vi "I2C_UI.vi"() -> ()   [LabVIEW 2023]
doc: "Main VI Of the Application that peroform the I2C Controller"
uses:
  Controls/Button.ctl
  Controls/Customized_Ring.ctl
  Controls/Add_Target_Specification_.ctl
  Controls/Queue_Operation.ctl
  Controls/State_and_Data.ctl
  Controls/I2C_Main_Data.ctl
  Class/I2C/I2C.lvclass
  Controls/Target_Data.ctl
  Controls/Text_File_Operation_Select.ctl
  Controls/UE_Driver_Operation_Select.ctl
  Controls/Converter_Operation_Select.ctl
  Controls/I2C_Data.ctl
  Class/I2C/Controls/Mode.ctl
  Drivers/Queue_Driver/QD_Main.vi
  SubVIs/I2C_to_Target_Spec.vi
  SubVIs/Target_Spec_To_I2C.vi
panel:
  in  "Configure":bool
  out "Tab Control":enum32{"Page 1", "Page 2"}(tab)
  out "Sample_Per_Us":dbl
  out "T_BUF":dbl
  out "T_HD_STA (uS)":dbl
  out "Off_Set (uS)":dbl
  out "Vmax":dbl
  out "Vmin":dbl
  in  "Read_Write":T1 items=["READ", "WRITE"]
  in  "Register_Name":T1
  in  "Target_Name":T1 items=["ADD TARGET"]
  out "Waveform Graph":waveform(dbl)[](graph)
  in  "Data Line":string
  out "History":string
  in  "Error_In":errorcluster
  out "Error_Out":errorcluster
  out "T_HD_DAT (uS)":dbl
  out "T_SU_DAT (uS)":dbl
  out "Frequency (kHz)":dbl
  out "T_SU_STO":dbl
  out "T_Off (uS)":dbl
  out "T_On (uS)":dbl
  in  "Mode":T2
  in  "Update":T2
  in  "Delete":T2
  in  "Target_Select":T1 items=["ADD TARGET"]
  out "Target_Specification":T3 {"Target_Address" format="%x"; "Target_Type" items=["10 Bit Address", "7 Bit Address"]; "T_On (uS)" min=1e-06; "T_Off (uS)" min=1e-06}
  in  "ADD":T2
  # "I2C CONTROLLER"
  # "Target Selection"
  # "History"
  # "Waveform data"
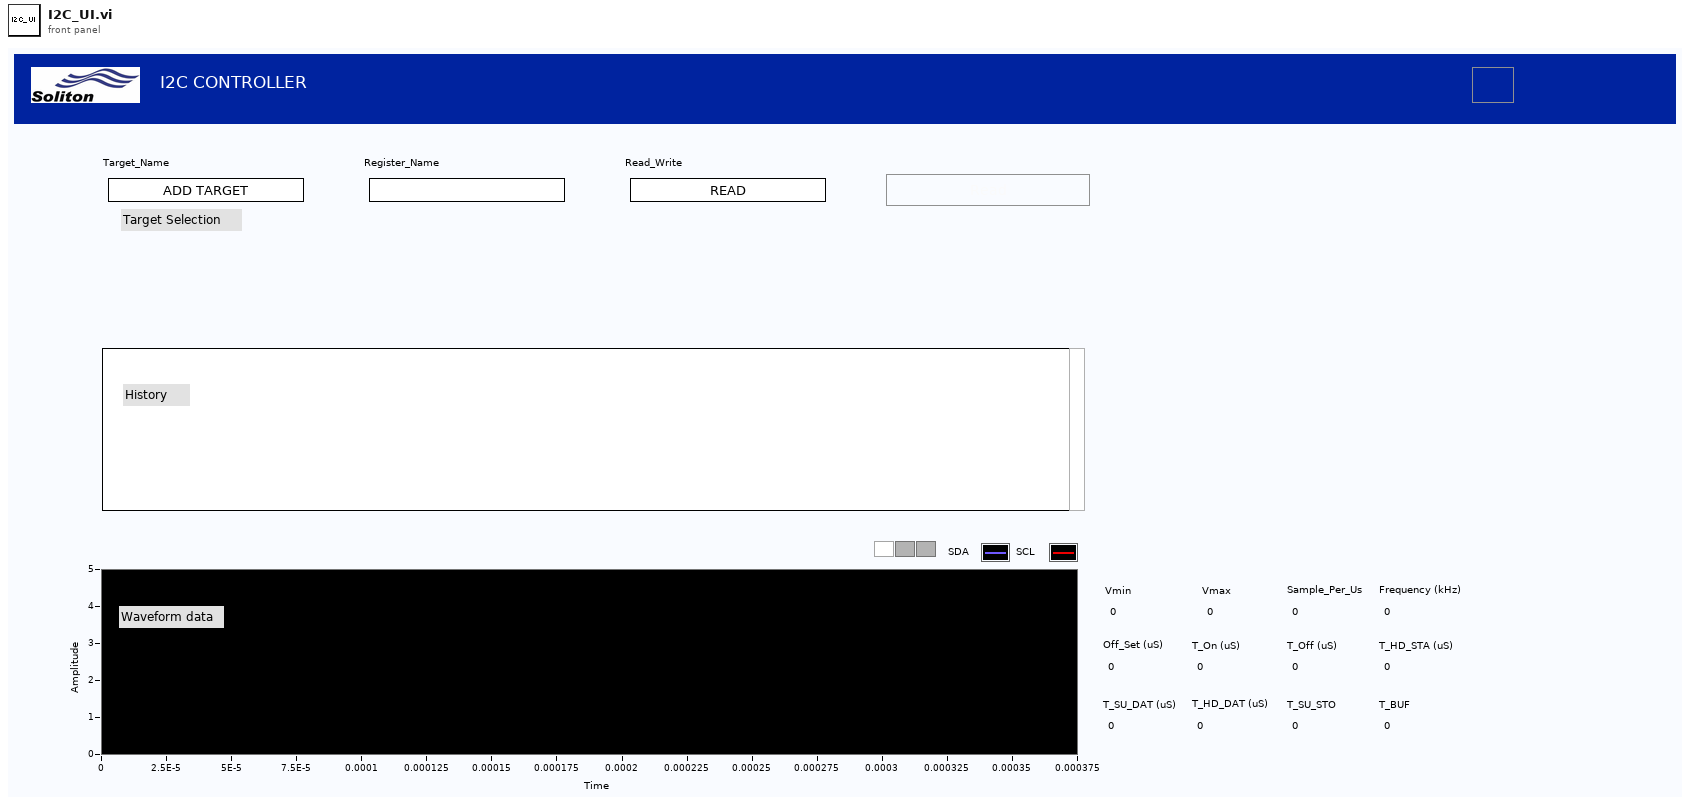
[diagram p1: front panel]
types:
  T1 = typedef "Customized_Ring.ctl" = u16
  T2 = typedef "Button.ctl" = bool
  T3 = typedef "Add_Target_Specification_.ctl" = cluster{"Target_Name":string, "Register_Name":string[], "Register_Address":u16[], "Vmin":dbl, "Vmax":dbl, "Off_Set (uS)":dbl, "T_HD_STA (uS)":dbl, "T_HD_DAT (uS)":dbl, "T_SU_DAT (uS)":dbl, "Frequency (kHz)":dbl, "T_SU_STO":dbl, "T_Off (uS)":dbl, "T_On (uS)":dbl, "T_BUF":dbl, "Sample_Per_Us":dbl, "Target_Type":T1, "Target_Address":u16}
  T4 = typedef "I2C_Main_Data.ctl" = cluster{"Target_Data":map{string, refnum<class "I2C.lvclass">}, "Class_Path":path, "Current_Page":enum32{"Page 1", "Page 2"}, "Class_Names":string[], "I2C_Class":refnum<class "I2C.lvclass">, "Target_Names":string[], "Register_Names":string[], "Selected_Target_Name":string, "Selected_Register_Name":string, "Target_Specification":T5, "Selected_Target_Config":string, "Read_Write":T1, "Add_Target_Reference":refnum<vi>, "Data_Line":string, "I2C_Waveform":waveform(dbl)[], "History":string, "Point_Target_Select":i32, "Ini_File_Path":path, "TVI_Reference":refnum<vi>, "vi reference":refnum<vi>}
  T5 = typedef "Target_Data.ctl" = cluster{"Target_Name":string, "Register_Name":string[], "Register_Address":u16[], "Vmin":dbl, "Vmax":dbl, "Off_Set (uS)":dbl, "T_HD_STA (uS)":dbl, "T_HD_DAT (uS)":dbl, "T_SU_DAT (uS)":dbl, "Frequency (kHz)":dbl, "T_SU_STO":dbl, "T_Off (uS)":dbl, "T_On (uS)":dbl, "T_BUF":dbl, "Sample_Per_Us":dbl, "Target_Type":T1, "Target_Address":u16}
  T6 = typedef "Queue_Operation.ctl" = enum16{"Obtain_Queue", "Enqueue", "Enqueue_First", "Enqueue_N", "Lossy_Enqueue", "Preview", "Queue_Status", "Dequeue", "Flush", "Release_Queue"}
  T7 = typedef "State_and_Data.ctl" = cluster{"State":string, "Data":variant}
  T8 = typedef "I2C_Data.ctl" = cluster{"Vmin":dbl, "Vmax":dbl, "Input":string, "Off_Set (uS)":dbl, "T_HD_STA (uS)":dbl, "Sample_Per_Us":dbl, "T_HD_DAT (uS)":dbl, "T_SU_DAT (uS)":dbl, "Frequency (kHz)":dbl, "T_SU_STO":dbl, "T_Off (uS)":dbl, "T_On (uS)":dbl, "T_BUF":dbl, "Target_Address":u16, "Selected_Register_Address":u8, "Byte_Array":u8[], "Target_Name":string, "Register_Name":string[], "Register_Address":u8[], "Target_Type":T1, "Register_Data":string[]}
  T9 = typedef "UE_Driver_Operation_Select.ctl" = enum16{"Create_UE", "Get_Refnum", "Generate_UE", "Destroy_UE"}
  T10 = typedef "Text_File_Operation_Select.ctl" = enum16{"Initialize", "Read", "Write"}
  T11 = typedef "Converter_Operation_Select.ctl" = enum16{"String_To_Data", "Data_to_String"}
  T12 = typedef "Mode.ctl" = enum16{"Read", "Write"}
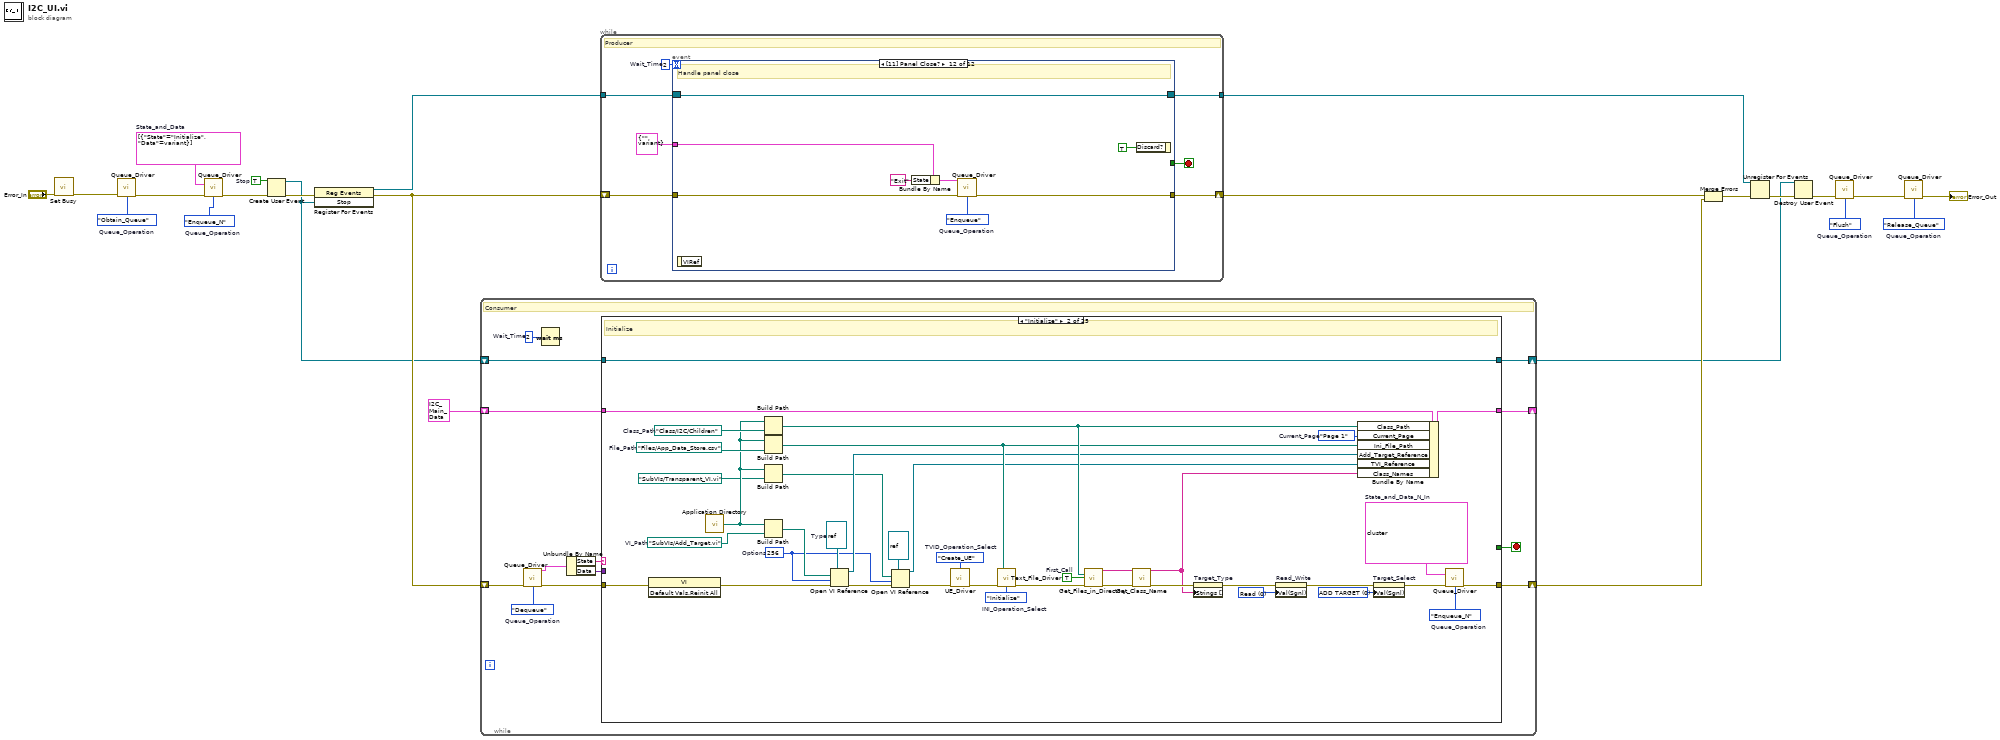
[diagram p0: block diagram]
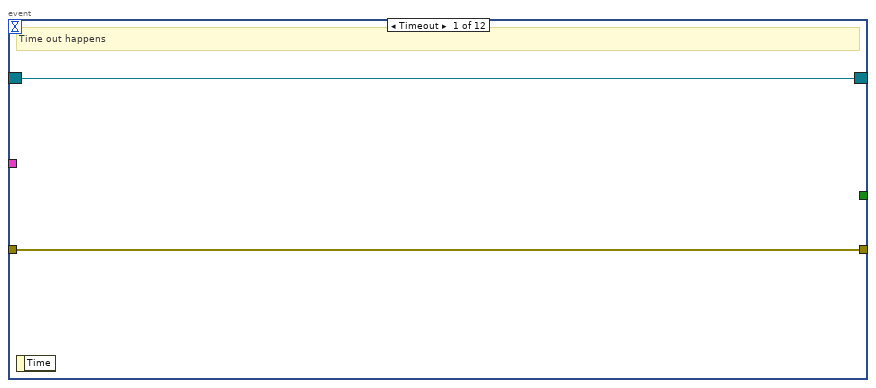
[diagram p2: hidden frame]
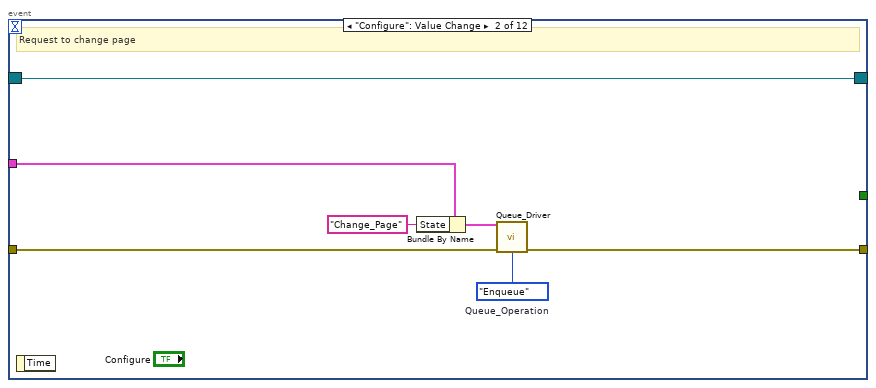
[diagram p3: hidden frame]
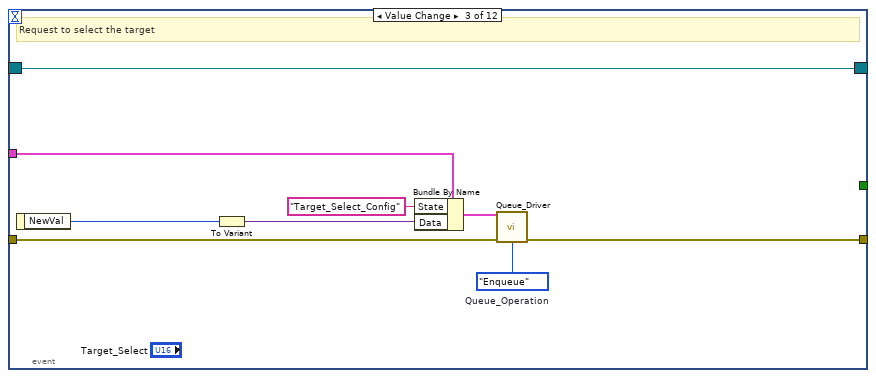
[diagram p4: hidden frame]
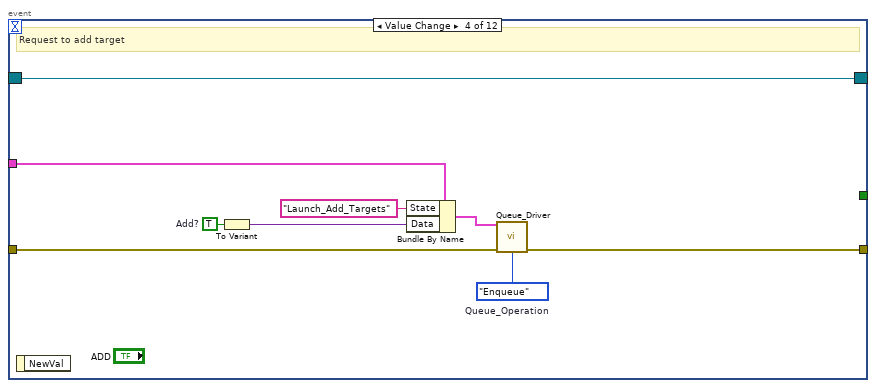
[diagram p5: hidden frame]
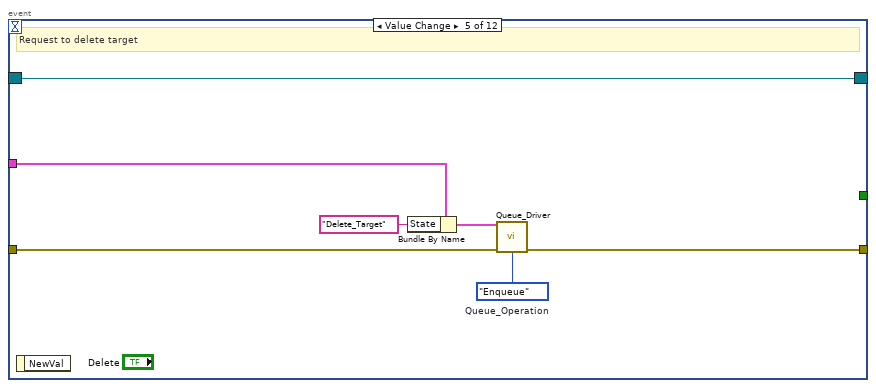
[diagram p6: hidden frame]
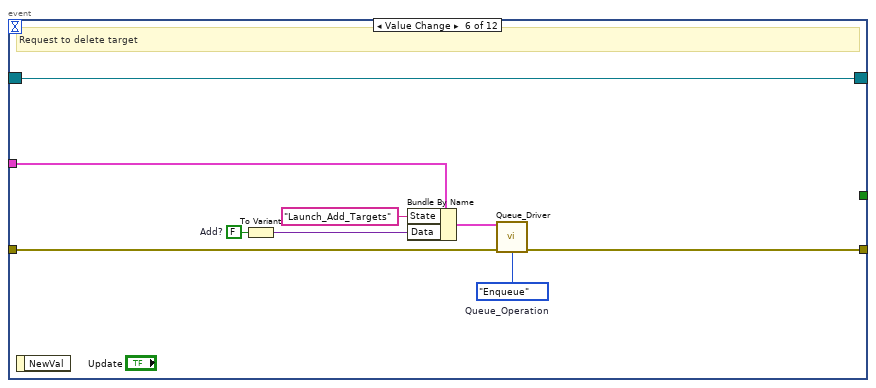
[diagram p7: hidden frame]
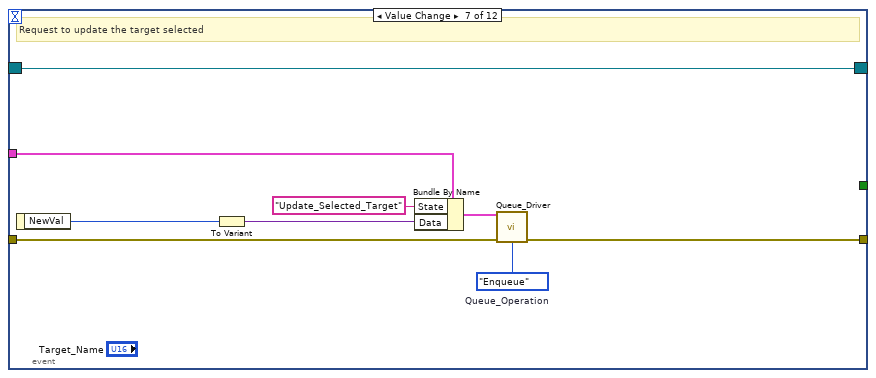
[diagram p8: hidden frame]
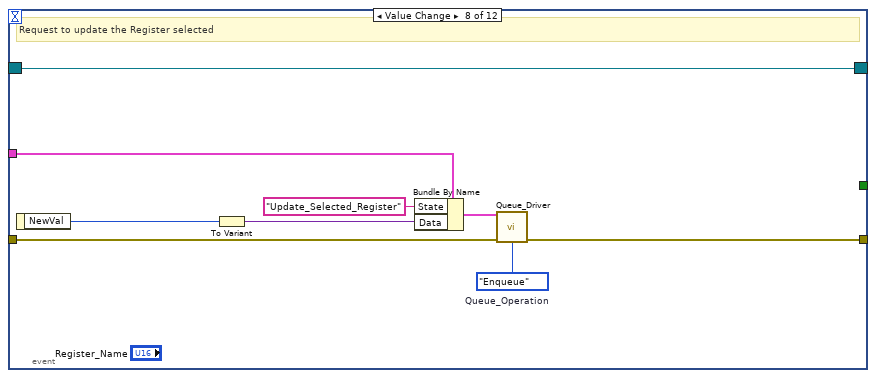
[diagram p9: hidden frame]
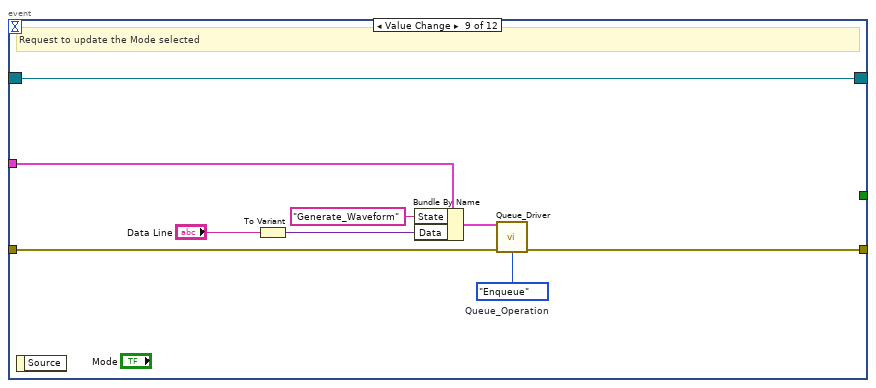
[diagram p10: hidden frame]
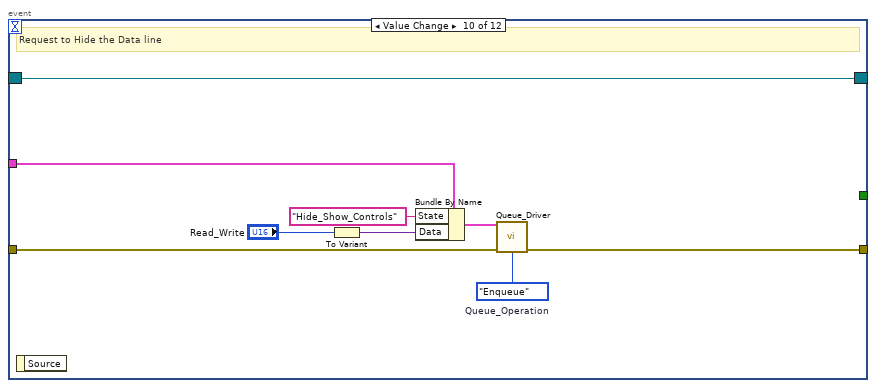
[diagram p11: hidden frame]
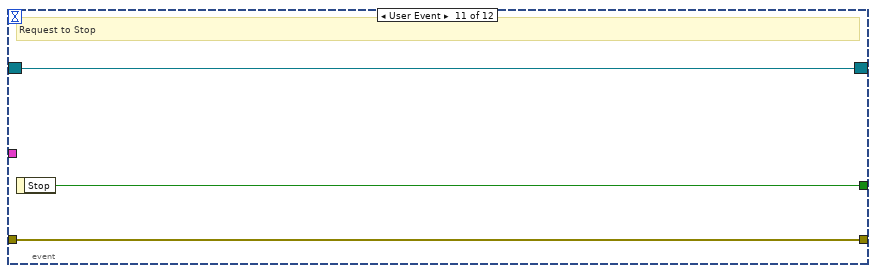
[diagram p12: hidden frame]
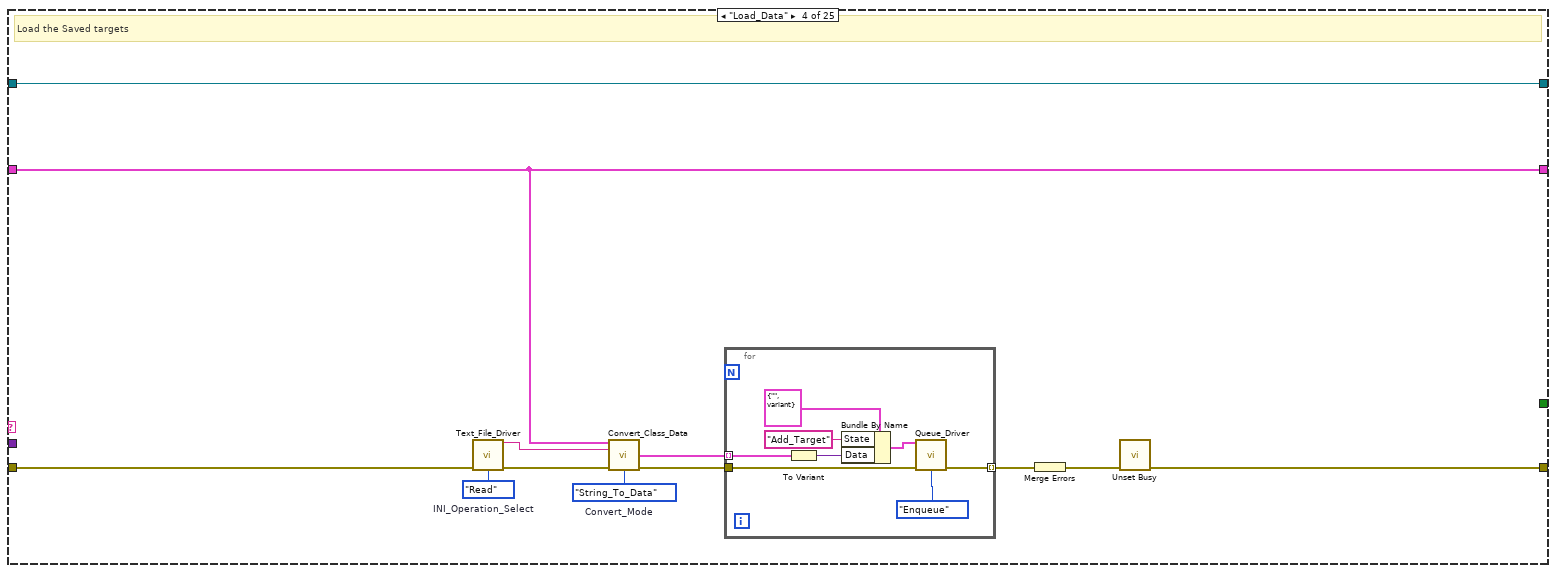
[diagram p15: hidden frame]
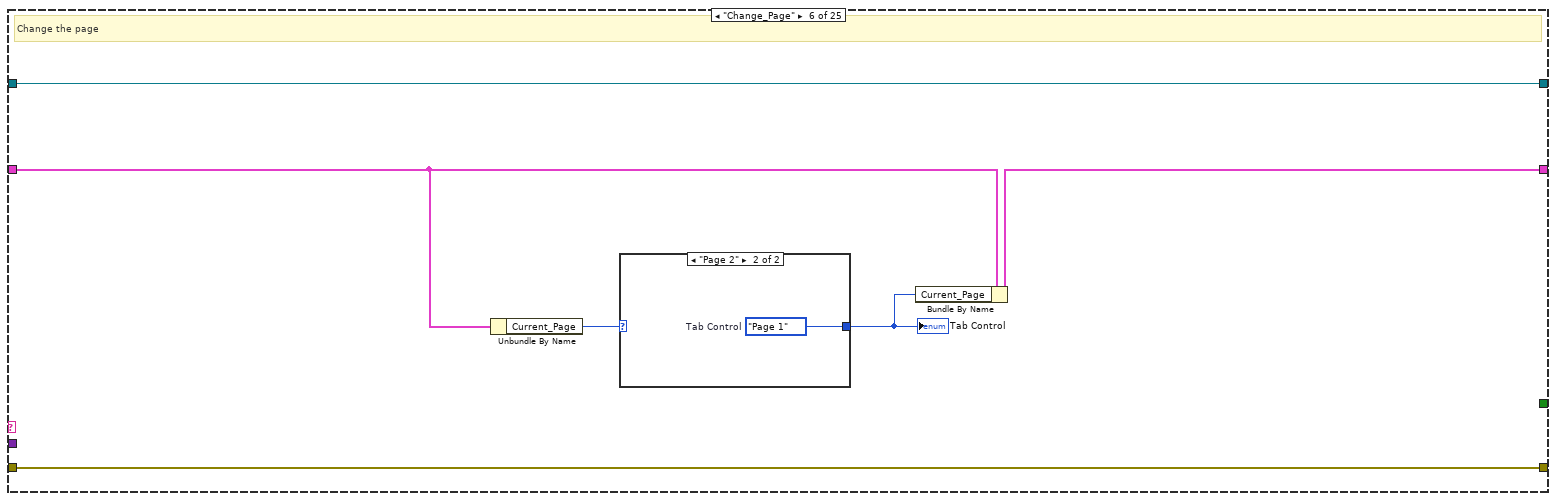
[diagram p17: hidden frame]
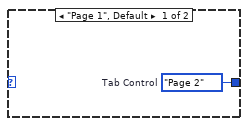
[diagram p18: hidden frame]
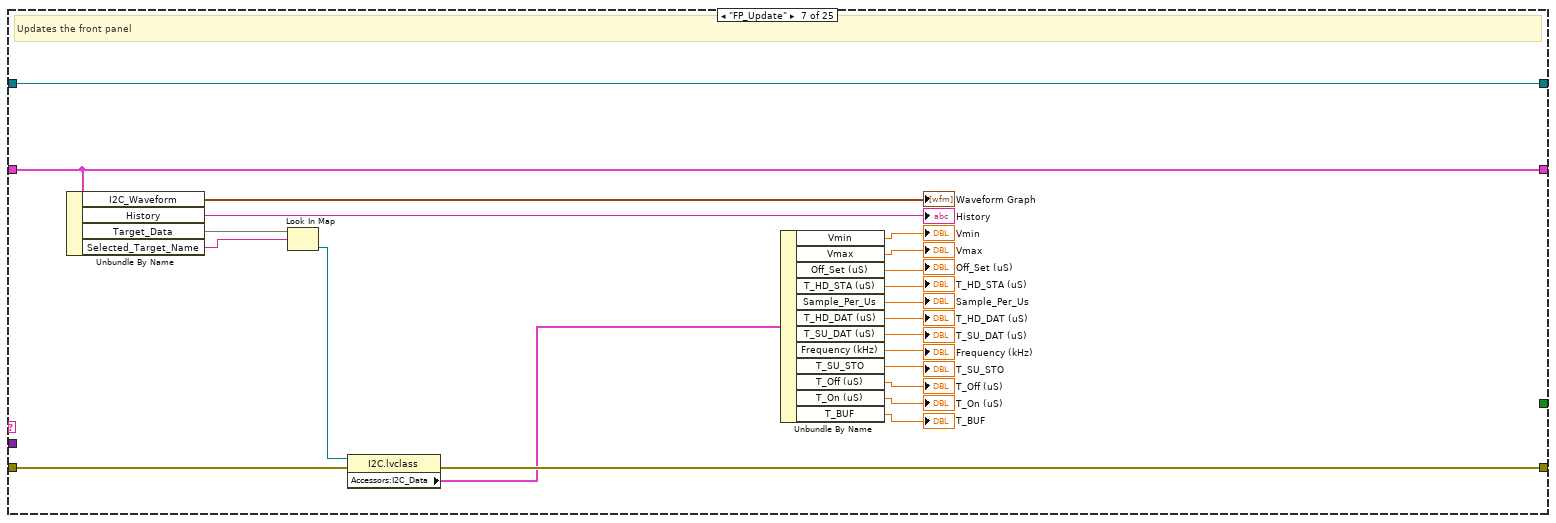
[diagram p19: hidden frame]
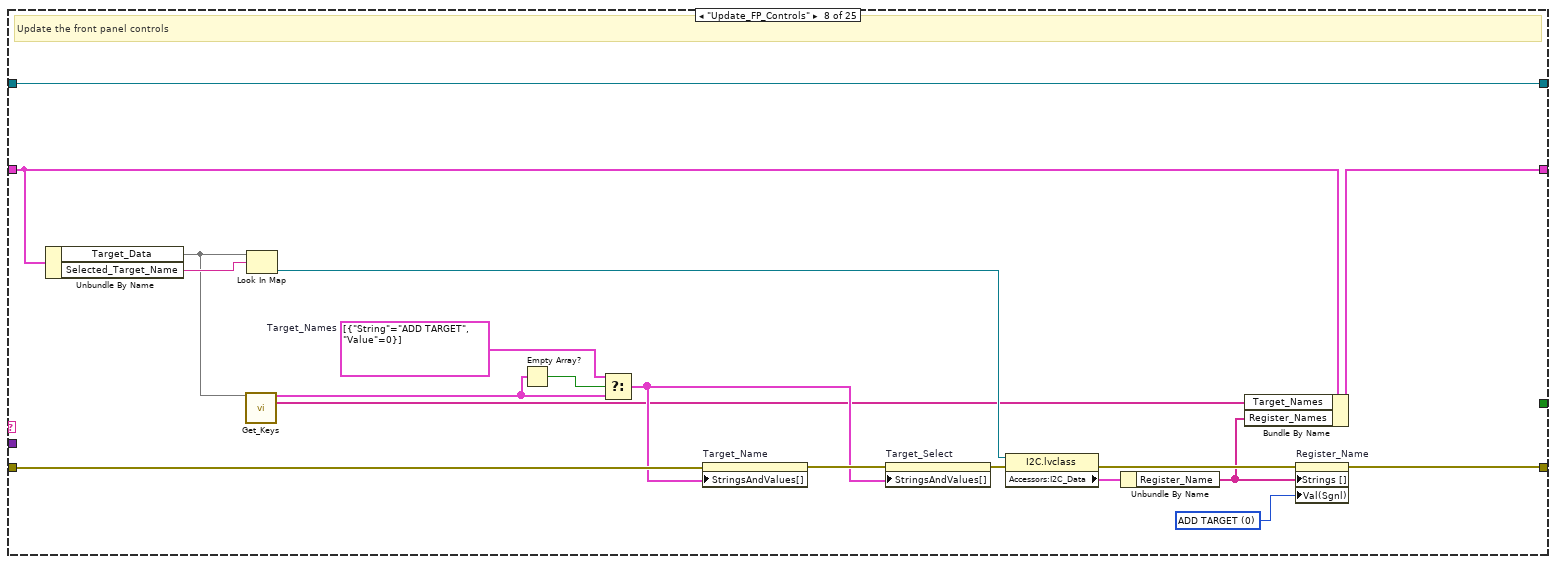
[diagram p20: hidden frame]
diagram:
  w8 = Queue_Operation."Release_Queue"  # Queue_Operation
  w9 = Queue_Operation."Flush"  # Queue_Operation
  w19 = TRUE  # Stop
  w3 = T7[] [{"State"="Initialize", "Data"=variant}]  # State_and_Data
  w22 = Queue_Operation."Enqueue_N"  # Queue_Operation
  w23 = Queue_Operation."Obtain_Queue"  # Queue_Operation
  n1 = call <vilib>:"Set Busy.vi"("error in (no error)"="Error_In") -> ("error out"=w1:errorcluster)  [unwired: 9 in, 1 out]
  n2 = call-poly "Queue_Driver.vi"("Error_In"=w1, "Queue_Operation"=w23) -> ("Error_Out"=w24:errorcluster)  [unwired: 11 in, 2 out]
  n3 = call-poly "Queue_Driver.vi"("State_and_Data_N_In"=w3, "Error_In"=w24, "Queue_Operation"=w22) -> ("Error_Out"=w7:errorcluster)  [unwired: 10 in, 2 out]
  n4 = Create User Event(user event datatype=w19, error in=w7) -> (user event=w4:refnum<user-event>, error out=w20:errorcluster)
  n5 = register-events(error in=w20, w4) -> (reference out=w18:refnum<event-registration>, error out=w5:errorcluster)  [unwired: 1 in]
  n6 = while {
    shift-right: [w29] -> w12
    shift-left: w4 -> [w30]
    shift-right: [w28] -> _
    shift-left: T4 {"Target_Data"={}, "Class_Path"=path "", "Current_Page"=enum."Page 1", "Class_Names"=[], "I2C_Class"=refnum, "Target_Names"=[], "Register_Names"=[], "Selected_Target_Name"="", "Selected_Register_Name"="", "Target_Specification"={"Target_Name"="", "Register_Name"=[], "Register_Address"=[], "Vmin"=0.0, "Vmax"=0.0, "Off_Set (uS)"=0.0, "T_HD_STA (uS)"=0.0, "T_HD_DAT (uS)"=0.0, "T_SU_DAT (uS)"=0.0, "Frequency (kHz)"=0.0, "T_SU_STO"=0.0, "T_Off (uS)"=0.0, "T_On (uS)"=0.0, "T_BUF"=0.0, "Sample_Per_Us"=0.0, "Target_Type"=0, "Target_Address"=0}, "Selected_Target_Config"="", "Read_Write"=0, "Add_Target_Reference"=refnum, "Data_Line"="", "I2C_Waveform"=[], "History"="", "Point_Target_Select"=0, "Ini_File_Path"=path "", "TVI_Reference"=refnum, "vi reference"=refnum} -> [w31]
    shift-right: [w27] -> w16
    shift-left: w5 -> [w37]
    stop <- w26 stop-if-true
    w25 = u32 2  # Wait_Time
    w35 = Queue_Operation."Dequeue"  # Queue_Operation
    # "Consumer"
    n7 = call-poly "Queue_Driver.vi"("Error_In"=w37, "Queue_Operation"=w35) -> ("State_and_Data_Out"=w34:T7, "Error_Out"=w36:errorcluster)  [unwired: 11 in, 1 out]
    n8 = Wait (ms)(milliseconds to wait=w25) -> ()  [unwired: 1 out]
    n9 = Unbundle By Name(w34) -> ("State"=w33:string, "Data"=w32:variant)
    n10 = case shown="\"Initialize\"" w33 {
      tunnel: [w40 w63 w82 w85 w105 w111 w128 w149 w160 w166 w179 w195 w222 w253 w271 w306 w314 w327 w342 w354 w364 w434 w440 w446 w452] -> w27
      tunnel: w36 -> [w40 w78 w82 w84 w105 w111 w135 w148 w161 w177 w192 w195 w201 w256 w279 w306 w326 w337 w351 w354 w367 w437 w440 w448 w461]
      tunnel: w32 -> [_ _ _ _ _ _ _ _ _ w176 _ _ w199 w249 _ _ w323 w334 w349 _ w362 _ _ w449 _]
      tunnel: w31 -> [w39 w56 w81 w89 w104 w109 w133 w153 w157 w175 w190 w194 w229 w252 w277 w305 w324 w335 w345 w353 w366 w435 w439 w447 w458]
      tunnel: [w39 w76 w81 w89 w104 w107 w133 w144 w157 w173 w190 w194 w226 w252 w275 w305 w319 w330 w344 w353 w368 w423 w439 w447 w457] -> w28
      tunnel: w30 -> [w38 w79 w80 w94 w103 w110 w134 w154 w163 w178 w191 w193 w230 w257 w278 w304 w325 w336 w350 w352 w369 w436 w438 w450 w464]
      tunnel: [w38 w79 w80 w94 w103 w110 w134 w154 w163 w178 w191 w193 w230 w257 w278 w304 w325 w336 w350 w352 w369 w436 w438 w450 w463] -> w29
      tunnel: [_ _ _ _ _ _ _ _ _ _ _ _ _ _ _ _ _ _ _ _ _ _ _ _ w462] -> w26
      frame Default {
      }
      frame "Initialize" {
        w41 = T1 0 items=["Read", "Write"] ("Value (Signaling)")
        w52 = UE_Driver_Operation_Select."Create_UE"  # TVID_Operation_Select
        w54 = TRUE  # First_Call
        w58 = T1 0 items=["ADD TARGET"] ("Value (Signaling)")
        w64 = T7[] [{"State"="Update_FP_Controls", "Data"=variant(cluster{"Current_Data":dbl, "Temp_Data":dbl} {"Current_Data"=0.0, "Temp_Data"=0.0})}, {"State"="Config_FP_Update", "Data"=variant(cluster{"Current_Data":dbl, "Temp_Data":dbl} {"Current_Data"=0.0, "Temp_Data"=0.0})}, {"State"="Load_Data", "Data"=variant(cluster{"Current_Data":dbl, "Temp_Data":dbl} {"Current_Data"=0.0, "Temp_Data"=0.0})}]  # State_and_Data_N_In
        w65 = Queue_Operation."Enqueue_N"  # Queue_Operation
        w67 = Text_File_Operation_Select."Initialize"  # INI_Operation_Select
        w68 = path "Files/App_Data_Store.csv"  # File_Path
        w69 = refnum<vi> refnum  # Type
        w43 = 256  # Options
        w72 = path "SubVIs/Add_Target.vi"  # VI_Path
        w74 = enum32{"Page 1", "Page 2"}."Page 1"  # Current_Page
        w77 = path "Class/I2C/Children"  # Class_Path
        # "Initialize"
        n11 = invoke class="VI" method="Default Vals.Reinit All"(error in=w78) -> (error out=w70:errorcluster)  [unwired: 2 in, 2 out]
        n12 = call <vilib>:"Application Directory.vi"() -> ("Application Directory"=w50:path)
        n13 = Build Path(base path=w50, name or relative path=w77) -> (appended path=w66:path)
        n14 = Build Path(base path=w50, name or relative path=w68) -> (appended path=w62:path)
        n15 = Build Path(base path=w50, name or relative path=path "SubVIs/Transparent_VI.vi") -> (appended path=w46:path)
        n16 = Build Path(base path=w50, name or relative path=w72) -> (appended path=w71:path)
        n17 = Open VI Reference(type specifier VI Refnum (for type only)=w69, vi path=w71, options=w43, error in (no error)=w70) -> (vi reference=w51:refnum<vi>, error out=w48:errorcluster)  [unwired: 2 in]
        n18 = Open VI Reference(type specifier VI Refnum (for type only)=refnum<vi> refnum, vi path=w46, options=w43, error in (no error)=w48) -> (vi reference=w44:refnum<vi>, error out=w47:errorcluster)  [unwired: 2 in]
        n19 = call "UE_Driver.vi"("TVID_Operation_Select"=w52, "Error_In"=w47) -> ("Error_Out"=w53:errorcluster)  [unwired: 11 in, 2 out]
        n20 = call "Text_File_Driver.vi"("Config_File_Path"=w62, "Error_Out"=w53, "INI_Operation_Select"=w67) -> ("Error_Out"=w57:errorcluster)  [unwired: 11 in, 1 out]
        n21 = call "Get_Files_in_Directory.vi"("File_Path"=w66, "First_Call"=w54, "Error_In"=w57) -> ("File_Names_Out"=w75:string[], "Error_Out"=w61:errorcluster)  [unwired: 11 in]
        n22 = call "Get_Class_Name.vi"("File_Names"=w75, "Error_In"=w61) -> ("Class_Names"=w60:string[], "Error_Out"=w73:errorcluster)  [unwired: 12 in]
        n23 = property on="Target_Type" class="Ring (strict)"(error in=w73, "Strings []"=w60) -> (error out=w55:errorcluster)  [unwired: 1 in, 1 out]
        n24 = property on="Read_Write" class="Ring (strict)"(error in=w55, "Val(Sgnl)"=w41) -> (error out=w42:errorcluster)  [unwired: 1 in, 1 out]
        n25 = Bundle By Name(cluster=w56, "Class_Path"=w66, "Current_Page"=w74, "Ini_File_Path"=w62, "Add_Target_Reference"=w51, "TVI_Reference"=w44, "Class_Names"=w60) -> (w76:T4)
        n26 = property on="Target_Select" class="Ring (strict)"(error in=w42, "Val(Sgnl)"=w58) -> (error out=w59:errorcluster)  [unwired: 1 in, 1 out]
        n27 = call-poly "Queue_Driver.vi"("State_and_Data_N_In"=w64, "Error_In"=w59, "Queue_Operation"=w65) -> ("Error_Out"=w63:errorcluster)  [unwired: 10 in, 2 out]
      }
      frame "---------------------Setup_States------------------" {
      }
      frame "Load_Data" {
        w90 = Converter_Operation_Select."String_To_Data"  # Convert_Mode
        w93 = Text_File_Operation_Select."Read"  # INI_Operation_Select
        # "Load the Saved targets"
        n28 = call "Text_File_Driver.vi"("Error_Out"=w84, "INI_Operation_Select"=w93) -> ("Data_Out"=w91:string, "Error_Out"=w92:errorcluster)  [unwired: 12 in]
        n29 = call "Convert_Class_Data.vi"("I2C_Data"=w89, "CSV_String_In"=w91, "Error_In"=w92, "Convert_Mode"=w90) -> ("Data"=w83:T8[], "Error_Out"=w87:errorcluster)  [unwired: 8 in, 2 out]
        n30 = for {
          tunnel: [w102] -> w88 mode=indexing
          tunnel: w83 -> [w98] mode=indexing
          tunnel: w87 -> [w95]
          n31 = To Variant(anything=w98) -> (Variant=w97:variant)
          n32 = Bundle By Name(cluster=T7 {"State"="", "Data"=variant} ("State_and_Data_In"), "State"="Add_Target", "Data"=w97) -> (w99:T7)
          n33 = call-poly "Queue_Driver.vi"("State_and_Data_In"=w99, "Error_In"=w95, "Queue_Operation"=Queue_Operation."Enqueue") -> ("Error_Out"=w102:errorcluster)  [unwired: 10 in, 2 out]
        }
        n34 = Merge Errors(w88) -> (w86:errorcluster)
        n35 = call <vilib>:"Unset Busy.vi"("error in (no error)"=w86) -> ("error out"=w85:errorcluster)  [unwired: 10 in]
      }
      frame "-----------------Front_Panel_Updates--------------" {
      }
      frame "Change_Page" {
        # "Change the page"
        n36 = Unbundle By Name(w109) -> ("Current_Page"=w108:enum32{"Page 1", "Page 2"})
        n37 = case shown="\"Page 2\"" w108 {
          tunnel: [w112 w113] -> w106
          frame "Page 1", Default {
            w112 = enum32{"Page 1", "Page 2"}."Page 2"  # Tab Control
          }
          frame "Page 2" {
            w113 = enum32{"Page 1", "Page 2"}."Page 1"  # Tab Control
          }
        }
        "Tab Control" <- w106
        n38 = Bundle By Name(cluster=w109, "Current_Page"=w106) -> (w107:T4)
      }
      frame "FP_Update" {
        # "Updates the front panel"
        n39 = Unbundle By Name(w133) -> ("I2C_Waveform"=→"Waveform Graph":waveform(dbl)[], "History"=→"History":string, "Target_Data"=w130:map{string, refnum<class "I2C.lvclass">}, "Selected_Target_Name"=w129:string)
        n40 = Look In Map(map=w130, key=w129) -> (value=w127:refnum<class "I2C.lvclass">)  [unwired: 1 in, 1 out]
        n41 = property class="I2C.lvclass"(reference=w127, error in=w135) -> (error out=w128:errorcluster, "Accessors:I2C_Data"=w126:T8)  [unwired: 1 out]
        n42 = Unbundle By Name(w126) -> ("Vmin"=→"Vmin":dbl, "Vmax"=→"Vmax":dbl, "Off_Set (uS)"=→"Off_Set (uS)":dbl, "T_HD_STA (uS)"=→"T_HD_STA (uS)":dbl, "Sample_Per_Us"=→"Sample_Per_Us":dbl, "T_HD_DAT (uS)"=→"T_HD_DAT (uS)":dbl, "T_SU_DAT (uS)"=→"T_SU_DAT (uS)":dbl, "Frequency (kHz)"=→"Frequency (kHz)":dbl, "T_SU_STO"=→"T_SU_STO":dbl, "T_Off (uS)"=→"T_Off (uS)":dbl, "T_On (uS)"=→"T_On (uS)":dbl, "T_BUF"=→"T_BUF":dbl)
      }
      frame "Update_FP_Controls" {
        w136 = T1 0 items=["ADD TARGET"] ("Value (Signaling)")
        w141 = cluster{"String":string, "Value":u16}[] [{"String"="ADD TARGET", "Value"=0}]  # Target_Names
        # "Update the front panel controls"
        n43 = Unbundle By Name(w153) -> ("Target_Data"=w140:map{string, refnum<class "I2C.lvclass">}, "Selected_Target_Name"=w146:string)
        n44 = call "Get_Keys.vi"("Target_Data"=w140) -> ("Keys_and_Index"=w139:cluster{"String":string, "Value":u16}[], "Keys"=w137:string[])  [unwired: 10 in, 3 out]
        n45 = Look In Map(map=w140, key=w146) -> (value=w151:refnum<class "I2C.lvclass">)  [unwired: 1 in, 1 out]
        n46 = Empty Array?(array=w139) -> (empty?=w142:bool)
        n47 = Select(t=w141, s=w142, f=w139) -> (s? t:f=w138:cluster{"String":string, "Value":u16}[])
        n48 = property on="Target_Name" class="Ring (strict)"(error in=w148, "StringsAndValues[]"=w138) -> (error out=w147:errorcluster)  [unwired: 1 in, 1 out]
        n49 = property on="Target_Select" class="Ring (strict)"(error in=w147, "StringsAndValues[]"=w138) -> (error out=w145:errorcluster)  [unwired: 1 in, 1 out]
        n50 = property class="I2C.lvclass"(reference=w151, error in=w145) -> (error out=w152:errorcluster, "Accessors:I2C_Data"=w150:T8)  [unwired: 1 out]
        n51 = Unbundle By Name(w150) -> ("Register_Name"=w143:string[])
        n52 = Bundle By Name(cluster=w153, "Target_Names"=w137, "Register_Names"=w143) -> (w144:T4)
        n53 = property on="Register_Name" class="Ring (strict)"(error in=w152, "Strings []"=w143, "Val(Sgnl)"=w136) -> (error out=w149:errorcluster)  [unwired: 1 in, 1 out]
      }
      frame "Config_FP_Update" {
        # "Updates the config panel display"
        n54 = Unbundle By Name(w157) -> ("Target_Data"=w158:map{string, refnum<class "I2C.lvclass">}, "Selected_Target_Config"=w159:string)
        n55 = Look In Map(map=w158, key=w159) -> (value=w162:refnum<class "I2C.lvclass">)  [unwired: 1 in, 1 out]
        n56 = property class="I2C.lvclass"(reference=w162, error in=w161) -> (error out=w160:errorcluster, "Accessors:I2C_Data"=w156:T8)  [unwired: 1 out]
        n57 = call-poly "Converter.vi"("I2C_Data"=w156) -> ("Target_Specification"=→"Target_Specification":T3)  [unwired: 14 in]
      }
      frame "Hide_Show_Controls" {
        w170 = "Write"  # Text
        w171 = "Read"  # Text
        # "Hide and show the data line in read and write mode respectively"
        n58 = Unbundle By Name(w175) -> ("Read_Write"=w174:T1)
        n59 = Variant To Data(error in=w177, type=w174, Variant=w176) -> (data=w168:T1, error out=w169:errorcluster)
        n60 = Bundle By Name(cluster=w175, "Read_Write"=w168) -> (w173:T4)
        n61 = Not Equal To 0?(x=w168) -> (x != 0?=w164:bool)
        n62 = property on="Data Line" class="Str"(error in=w169, "Visible"=w164, "Value"="", "Key Focus"=w164) -> (error out=w167:errorcluster)  [unwired: 1 in, 1 out]
        n63 = Select(t=w170, s=w164, f=w171) -> (s? t:f=w172:string)
        n64 = property on="Mode" class="Bool (strict)"(error in=w167, "BoolText.Text"=w172) -> (error out=w166:errorcluster)  [unwired: 1 in, 1 out]
      }
      frame "Point_Target_Select" {
        w185 = T1 0 items=["ADD TARGET"]  # Type
        w188 = 0  # Index
        # "Makes the controls point valid values"
        n65 = Unbundle By Name(w190) -> ("Selected_Target_Name"=w182:string, "Target_Data"=w183:map{string, refnum<class "I2C.lvclass">})  [unwired: 1 out]
        n66 = call "Get_Keys.vi"("Target_Data"=w183) -> ("Keys"=w181:string[])  [unwired: 10 in, 4 out]
        n67 = Search 1D Array(1D array=w181, element=w182) -> (index of element=w180:i32)  [unwired: 1 in]
        n68 = Greater Or Equal To 0?(x=w180) -> (x >= 0?=w187:bool)
        n69 = Select(t=w180, s=w187, f=w188) -> (s? t:f=w186:i32)
        n70 = Coerce To Type(0:w186, 1:w185) -> (2:w184:T1)
        n71 = property on="Target_Select" class="Ring (strict)"(error in=w192, "Val(Sgnl)"=w184) -> (error out=w189:errorcluster)  [unwired: 1 in, 1 out]
        n72 = property on="Target_Name" class="Ring (strict)"(error in=w189, "Val(Sgnl)"=w184) -> (error out=w179:errorcluster)  [unwired: 1 in, 1 out]
      }
      frame "--------------------Manage_Targets---------------" {
      }
      frame "Add_Target" {
        w206 = T7[] [{"State"="Update_FP_Controls", "Data"=variant(cluster{"Current_Data":dbl, "Temp_Data":dbl} {"Current_Data"=0.0, "Temp_Data"=0.0})}, {"State"="Config_FP_Update", "Data"=variant(cluster{"Current_Data":dbl, "Temp_Data":dbl} {"Current_Data"=0.0, "Temp_Data"=0.0})}, {"State"="Point_Target_Select", "Data"=variant(cluster{"Current_Data":dbl, "Temp_Data":dbl} {"Current_Data"=0.0, "Temp_Data"=0.0})}]  # State_and_Data_N_In
        w207 = Queue_Operation."Enqueue_N"  # Queue_Operation
        w208 = 0  # Type
        w221 = "%s\\\\%s\\\\%s.lvclass"  # Format_String
        # "Add targets and populate into controls"
        n73 = Unbundle By Name(w229) -> ("Target_Names"=w224:string[], "Target_Data"=w225:map{string, refnum<class "I2C.lvclass">}, "I2C_Class"=w227:refnum<class "I2C.lvclass">, "Class_Path"=w228:path, "Class_Names"=w223:string[])
        n74 = Variant To Data(error in=w201, type=T8 {"Vmin"=0.0, "Vmax"=1.0, "Input"="", "Off_Set (uS)"=0.0, "T_HD_STA (uS)"=0.0, "Sample_Per_Us"=0.0, "T_HD_DAT (uS)"=0.0, "T_SU_DAT (uS)"=0.0, "Frequency (kHz)"=0.0, "T_SU_STO"=0.0, "T_Off (uS)"=0.0, "T_On (uS)"=0.0, "T_BUF"=0.0, "Target_Address"=0, "Selected_Register_Address"=0, "Byte_Array"=[], "Target_Name"="", "Register_Name"=[], "Register_Address"=[], "Target_Type"=0, "Register_Data"=[]} ("I2C_Data"), Variant=w199) -> (data=w197:T8, error out=w200:errorcluster)
        n75 = Unbundle By Name(w197) -> ("Register_Name"=w198:string[], "Target_Name"=w205:string, "Target_Type"=w211:T1)
        n76 = Coerce To Type(0:w211, 1:w208) -> (2:w209:i32)
        n77 = Index Array(array=w223, index=w209) -> (element=w210:string)
        n78 = Format Into String(format string=w221, error in=w200, w228, w210, w210) -> (resulting string=w220:string, error out=w219:errorcluster)  [unwired: 1 in]
        n79 = String To Path(string=w220) -> (path=w217:path)
        n80 = call <vilib>:"Get LV Class Default Value.vi"("error in (no error)"=w219, "class path"=w217) -> ("error out"=w218:errorcluster, "object"=w215:refnum<class>)  [unwired: 8 in]
        n81 = To More Specific Class(target class=w227, reference=w215, error in=w218) -> (specific class reference=w214:refnum<class "I2C.lvclass">, error out=w216:errorcluster)
        n82 = property class="I2C.lvclass"(reference=w214, error in=w216, "Accessors:I2C_Data"=w197) -> (reference out=w212:refnum<class "I2C.lvclass">, error out=w203:errorcluster)
        n83 = Insert Into Array(array=w224, new element=w205) -> (w202:string[])  [unwired: 1 in]
        n84 = Insert Into Map(map in=w225, key=w205, value=w212) -> (map out=w213:map{string, refnum<class "I2C.lvclass">})  [unwired: 2 out]
        n85 = Index Array(array=w198) -> (element=w204:string)  [unwired: 1 in]
        n86 = Bundle By Name(cluster=w229, "Selected_Target_Name"=w205, "Target_Names"=w202, "Selected_Target_Config"=w205, "Target_Data"=w213, "Selected_Register_Name"=w204) -> (w226:T4)
        n87 = call-poly "Queue_Driver.vi"("State_and_Data_N_In"=w206, "Error_In"=w203, "Queue_Operation"=w207) -> ("Error_Out"=w222:errorcluster)  [unwired: 10 in, 2 out]
      }
      frame "Launch_Add_Targets" {
        w232 = UE_Driver_Operation_Select."Generate_UE"  # TVID_Operation_Select
        w242 = T8 {"Vmin"=0.0, "Vmax"=5.0, "Input"="", "Off_Set (uS)"=10.0, "T_HD_STA (uS)"=5.0, "Sample_Per_Us"=1000.0, "T_HD_DAT (uS)"=5.0, "T_SU_DAT (uS)"=0.25, "Frequency (kHz)"=0.0, "T_SU_STO"=4.0, "T_Off (uS)"=5.0, "T_On (uS)"=5.0, "T_BUF"=5.0, "Target_Address"=0, "Selected_Register_Address"=0, "Byte_Array"=[], "Target_Name"="", "Register_Name"=[], "Register_Address"=[], "Target_Type"=0, "Register_Data"=[]}  # Empty_I2C
        # "Launch the add target page to add or edit the targets"
        n88 = Unbundle By Name(w252) -> ("Add_Target_Reference"=w238:refnum<vi>, "TVI_Reference"=w234:refnum<vi>, "Target_Data"=w247:map{string, refnum<class "I2C.lvclass">}, "Selected_Target_Name"=w246:string)
        n89 = Variant To Data(error in=w256, type=FALSE, Variant=w249) -> (data=w243:bool, error out=w250:errorcluster)
        n90 = Look In Map(map=w247, key=w246) -> (value=w245:refnum<class "I2C.lvclass">)  [unwired: 1 in, 1 out]
        n91 = property class="I2C.lvclass"(reference=w245, error in=w250) -> (error out=w237:errorcluster, "Accessors:I2C_Data"=w244:T8)  [unwired: 1 out]
        n92 = Select(t=w242, s=w243, f=w244) -> (s? t:f=w240:T8)
        n93 = call-poly "Converter.vi"("I2C_Data"=w240) -> ("Target_Specification"=w231:T3)  [unwired: 14 in]
        n94 = call-by-ref "Start Asynchronous Call"(reference=w234, error in=w237) -> (error out=w235:errorcluster)  [unwired: 19 in, 2 out]
        n95 = call-by-ref "?"(reference=w238, error in=w235, "Data"=w231) -> (error out=w236:errorcluster, "Target_Specification_Out"=w239:T3, "Add?"=w251:bool, "Error_Out"=w254:errorcluster)  [unwired: 12 in, 1 out]
        n96 = call "UE_Driver.vi"("TVID_Operation_Select"=w232, "Error_In"=w236) -> ("Error_Out"=w233:errorcluster)  [unwired: 11 in, 2 out]
        n97 = Merge Errors(w233, w254) -> (w255:errorcluster)
        n98 = call-poly "Converter.vi"("Input_Data"=w239) -> ("I2C_Data"=w241:T8)  [unwired: 14 in]
        n99 = case shown="False" w251 {
          tunnel: w255 -> [w265 w266]
          tunnel: [w264 w266] -> w253
          tunnel: w241 -> [w259 _]
          frame False {
            w263 = Queue_Operation."Enqueue"  # Queue_Operation
            # "Add if added"
            n100 = To Variant(anything=w259) -> (Variant=w258:variant)
            n101 = Bundle By Name(cluster=T7 {"State"="", "Data"=variant} ("State_and_Data_In"), "State"="Add_Target", "Data"=w258) -> (w261:T7)
            n102 = call-poly "Queue_Driver.vi"("State_and_Data_In"=w261, "Error_In"=w265, "Queue_Operation"=w263) -> ("Error_Out"=w264:errorcluster)  [unwired: 10 in, 2 out]
          }
          frame True {
            # "Dont add if canceled"
          }
        }
      }
      frame "Delete_Target" {
        w272 = "%s"  # Format_String
        w274 = "Do you want to delete "  # Initial_Message
        # "Delete the targets"
        n103 = Unbundle By Name(w277) -> ("Target_Names"=w269:string[], "Target_Data"=w276:map{string, refnum<class "I2C.lvclass">}, "Selected_Target_Config"=w273:string)
        n104 = Empty Array?(array=w269) -> (empty?=w268:bool)
        n105 = Format Into String(format string=w272, initial string=w274, error in=w279, w273) -> (resulting string=w267:string, error out=w270:errorcluster)
        n106 = case shown="False" w268 {
          tunnel: w277 -> [w283 w303]
          tunnel: w276 -> [w299 _]
          tunnel: [w284 w303] -> w275
          tunnel: w273 -> [w294 _]
          tunnel: [w296 w302] -> w271
          tunnel: w270 -> [w290 w302]
          tunnel: w267 -> [w286 _]
          frame False {
            w288 = "No"  # Dont
            w287 = "Yes"  # Delete
            w291 = T7[] [{"State"="Update_FP_Controls", "Data"=variant(cluster{"Current_Data":dbl, "Temp_Data":dbl} {"Current_Data"=0.0, "Temp_Data"=0.0})}, {"State"="Point_Target_Select", "Data"=variant(cluster{"Current_Data":dbl, "Temp_Data":dbl} {"Current_Data"=0.0, "Temp_Data"=0.0})}, {"State"="Config_FP_Update", "Data"=variant(cluster{"Current_Data":dbl, "Temp_Data":dbl} {"Current_Data"=0.0, "Temp_Data"=0.0})}]  # State_and_Data_N_In
            w295 = Queue_Operation."Enqueue_N"  # Queue_Operation
            # "Delete if target exist"
            n107 = Unbundle By Name(w283) -> ("Target_Names"=w293:string[])
            n108 = Remove From Map(10:w294, 11:w299) -> (3:w297:map{string, refnum<class "I2C.lvclass">})  [unwired: 2 out]
            n109 = Search 1D Array(1D array=w293, element=w294) -> (index of element=w289:i32)  [unwired: 1 in]
            n110 = Two Button Dialog(message=w286, 1:w288, 2:w287) -> (T button?=w282:bool)
            n111 = Delete From Array(array=w293, index=w289) -> (array with subset deleted=w292:string[])  [unwired: 1 in, 1 out]
            n112 = Bundle By Name(cluster=w283, "Target_Names"=w292, "Target_Data"=w297) -> (w298:T4)
            n113 = Not(x=w282) -> (.not. x?=w280:bool)
            n114 = Select(t=w283, s=w280, f=w298) -> (s? t:f=w284:T4)
            n115 = Select(t=T7[] [] ("f"), s=w280, f=w291) -> (s? t:f=w285:T7[])
            n116 = call-poly "Queue_Driver.vi"("State_and_Data_N_In"=w285, "Error_In"=w290, "Queue_Operation"=w295) -> ("Error_Out"=w296:errorcluster)  [unwired: 10 in, 2 out]
          }
          frame True {
            w300 = "Ok"  # Ack
            w301 = "No targets to delete"  # Message
            # "Prompt user if there is no target"
            n117 = One Button Dialog(message=w301, button name ("OK")=w300) -> ()  [unwired: 1 out]
          }
        }
      }
      frame "----------------- Manage_States_Data---------------" {
      }
      frame "Update_Selected_Target" {
        w316 = Queue_Operation."Enqueue"  # Queue_Operation
        w317 = T7 {"State"="Update_FP_Controls", "Data"=variant}  # State_and_Data_In
        w322 = u16 0  # Type
        # "Update selected target"
        n118 = Unbundle By Name(w324) -> ("Target_Data"=w313:map{string, refnum<class "I2C.lvclass">}, "Target_Names"=w321:string[])
        n119 = Variant To Data(error in=w326, type=w322, Variant=w323) -> (data=w320:u16, error out=w315:errorcluster)
        n120 = To Long Integer(number=w320) -> (32bit integer=w318:i32)
        n121 = Index Array(array=w321, index=w318) -> (element=w312:string)
        n122 = Look In Map(map=w313, key=w312) -> (value=w310:refnum<class "I2C.lvclass">)  [unwired: 1 in, 1 out]
        n123 = property class="I2C.lvclass"(reference=w310, error in=w315) -> (error out=w311:errorcluster, "Accessors:I2C_Data"=w309:T8)  [unwired: 1 out]
        n124 = Unbundle By Name(w309) -> ("Register_Name"=w308:string[])
        n125 = Index Array(array=w308) -> (element=w307:string)  [unwired: 1 in]
        n126 = Bundle By Name(cluster=w324, "Selected_Target_Name"=w312, "Selected_Register_Name"=w307) -> (w319:T4)
        n127 = call-poly "Queue_Driver.vi"("State_and_Data_In"=w317, "Error_In"=w311, "Queue_Operation"=w316) -> ("Error_Out"=w314:errorcluster)  [unwired: 10 in, 2 out]
      }
      frame "Update_Selected_Register" {
        w333 = u16 0  # Type
        # "Update selected Register"
        n128 = Unbundle By Name(w335) -> ("Register_Names"=w332:string[])
        n129 = Variant To Data(error in=w337, type=w333, Variant=w334) -> (data=w331:u16, error out=w327:errorcluster)
        n130 = To Long Integer(number=w331) -> (32bit integer=w328:i32)
        n131 = Index Array(array=w332, index=w328) -> (element=w329:string)
        n132 = Bundle By Name(cluster=w335, "Selected_Register_Name"=w329) -> (w330:T4)
      }
      frame "Target_Select_Config" {
        w340 = Queue_Operation."Enqueue"  # Queue_Operation
        w341 = T7 {"State"="Config_FP_Update", "Data"=variant}  # State_and_Data_In
        w348 = 0  # Type
        # "Update selected target in config page"
        n133 = Unbundle By Name(w345) -> ("Target_Data"=w339:map{string, refnum<class "I2C.lvclass">})
        n134 = Variant To Data(error in=w351, type=w348, Variant=w349) -> (data=w347:i32, error out=w346:errorcluster)
        n135 = call "Get_Keys.vi"("Target_Data"=w339) -> ("Keys"=w338:string[])  [unwired: 10 in, 4 out]
        n136 = Index Array(array=w338, index=w347) -> (element=w343:string)
        n137 = Bundle By Name(cluster=w345, "Selected_Target_Config"=w343) -> (w344:T4)
        n138 = call-poly "Queue_Driver.vi"("State_and_Data_In"=w341, "Error_In"=w346, "Queue_Operation"=w340) -> ("Error_Out"=w342:errorcluster)  [unwired: 10 in, 2 out]
      }
      frame "---------------------I2C_Handling-------------------" {
      }
      frame "Generate_Waveform" {
        w361 = ""  # Data_Type
        # "Genearte waveforms"
        n139 = Unbundle By Name(w366) -> ("Target_Data"=w357:map{string, refnum<class "I2C.lvclass">}, "Selected_Target_Name"=w358:string, "Selected_Register_Name"=w356:string, "Read_Write"=w360:T1)
        n140 = Variant To Data(error in=w367, type=w361, Variant=w362) -> (data=w355:string, error out=w363:errorcluster)
        n141 = Look In Map(map=w357, key=w358) -> (key not found?=w359:bool, value=w365:refnum<class "I2C.lvclass">)  [unwired: 1 in]
        n142 = case shown="False" w359 {
          tunnel: [w404 w408] -> w368
          tunnel: w366 -> [w402 w408]
          tunnel: w365 -> [w401 _]
          tunnel: w356 -> [w376 _]
          tunnel: [w387 w407] -> w364
          tunnel: w363 -> [w385 w407]
          tunnel: w355 -> [w375 _]
          tunnel: w360 -> [w371 _]
          tunnel: w358 -> [w380 _]
          tunnel: w357 -> [w381 _]
          frame False {
            w382 = T7[] [{"State"="Update_History", "Data"=variant(cluster{"Current_Data":dbl, "Temp_Data":dbl} {"Current_Data"=0.0, "Temp_Data"=0.0})}, {"State"="FP_Update", "Data"=variant(cluster{"Current_Data":dbl, "Temp_Data":dbl} {"Current_Data"=0.0, "Temp_Data"=0.0})}]  # State_and_Data_N_In
            w383 = Mode."Read"  # Mode
            w386 = Queue_Operation."Enqueue_N"  # Queue_Operation
            # "Generate waveform"
            n143 = property class="I2C.lvclass"(reference=w401, error in=w385) -> (reference out=w388:refnum<class "I2C.lvclass">, error out=w397:errorcluster, "Accessors:I2C_Data"=w389:T8)
            n144 = Equal To 0?(x=w371) -> (x = 0?=w370:bool)
            n145 = Unbundle By Name(w389) -> ("Target_Address"=w393:u16, "Register_Address"=w395:u8[], "Register_Name"=w396:string[], "Register_Data"=w372:string[])
            n146 = Type Cast(type=w383, x=w371) -> (*(type *) &x=w384:T12)
            n147 = Search 1D Array(1D array=w396, element=w376) -> (index of element=w377:i32)  [unwired: 1 in]
            n148 = Replace Array Subset(array=w372, new element=w375, index=w377) -> (w374:string[])
            n149 = Index Array(array=w395, index=w377) -> (element=w394:u8)
            n150 = Select(t=w372, s=w370, f=w374) -> (s? t:f=w373:string[])
            n151 = Bundle By Name(cluster=w389, "Target_Address"=w393, "Selected_Register_Address"=w394, "Register_Data"=w373, "Input"=w375) -> (w398:T8)
            n152 = property class="I2C.lvclass"(reference=w388, error in=w397, "Accessors:I2C_Data"=w398) -> (reference out=w392:refnum<class "I2C.lvclass">, error out=w399:errorcluster)
            n153 = call-dynamic "Generate_I2C.vi"("Error_In"=w399, "Mode"=w384, "I2C in"=w392) -> ("Error_Out"=w400:errorcluster, "I2C out"=w391:refnum<class "I2C.lvclass">)  [unwired: 7 in]
            n154 = property class="I2C.lvclass"(reference=w391, error in=w400) -> (reference out=w379:refnum<class "I2C.lvclass">, error out=w403:errorcluster, "Accessors:I2C_Waveform"=w390:waveform(dbl)[])
            n155 = Insert Into Map(map in=w381, key=w380, value=w379) -> (map out=w378:map{string, refnum<class "I2C.lvclass">})  [unwired: 2 out]
            n156 = Bundle By Name(cluster=w402, "Target_Data"=w378, "I2C_Waveform"=w390) -> (w404:T4)
            n157 = call-poly "Queue_Driver.vi"("State_and_Data_N_In"=w382, "Error_In"=w403, "Queue_Operation"=w386) -> ("Error_Out"=w387:errorcluster)  [unwired: 10 in, 2 out]
          }
          frame True {
            w405 = "Ok"  # Acko
            w406 = "Please add targets to sent or receive data"  # Message
            # "Prompt user if no targets to send or receive the data"
            n158 = One Button Dialog(message=w406, button name ("OK")=w405) -> ()  [unwired: 1 out]
          }
        }
      }
      frame "Update_History" {
        w424 = "%s %s; %s %s; %s %s; %s %s; %s %s;\\n%s"  # Format_String
        w421 = "Time : "  # History_Data
        # "Update the history"
        n159 = Unbundle By Name(w435) -> ("Selected_Target_Name"=w418:string, "Selected_Register_Name"=w413:string, "Read_Write"=w430:T1, "Target_Data"=w419:map{string, refnum<class "I2C.lvclass">}, "History"=w409:string)
        n160 = Look In Map(map=w419, key=w418) -> (value=w416:refnum<class "I2C.lvclass">)  [unwired: 1 in, 1 out]
        n161 = property class="I2C.lvclass"(reference=w416, error in=w437) -> (error out=w417:errorcluster, "Accessors:I2C_Data"=w415:T8)  [unwired: 1 out]
        n162 = Unbundle By Name(w415) -> ("Register_Data"=w412:string[], "Register_Name"=w414:string[])
        n163 = Equal To 0?(x=w430) -> (x = 0?=w426:bool)
        n164 = Search 1D Array(1D array=w414, element=w413) -> (index of element=w411:i32)  [unwired: 1 in]
        n165 = Index Array(array=w412, index=w411) -> (element=w410:string)
        n166 = Format Date/Time String() -> (date/time string=w420:string)  [unwired: 3 in]
        n167 = Select(t="Read" ("input 7"), s=w426, f="Write" ("input 7")) -> (s? t:f=w427:string)
        n168 = Format Into String(format string=w424, error in=w417, w421, w420, "Target Name : " ("input 1"), w418, "Register Name : " ("input 3"), w413, "Mode : " ("input 7"), w427, "Data : " ("input 9"), w410, w409) -> (resulting string=w422:string, error out=w434:errorcluster)  [unwired: 1 in]
        n169 = Bundle By Name(cluster=w435, "History"=w422) -> (w423:T4)
      }
      frame "-----------------Exception_and_Exit----------------" {
      }
      frame "Error" {
        w445 = Queue_Operation."Enqueue"  # Queue_Operation
        # "Handle error"
        n170 = Variant To Data(error in=w448, type=w448, Variant=w449) -> (data=w442:errorcluster, error out=w444:errorcluster)
        n171 = call "Analyse_Error.vi"("Erroe_Under_Analyse"=w442, "Error_In"=w444) -> ("State_and_Data"=w441:T7, "Error_Out"=w443:errorcluster)  [unwired: 12 in]
        n172 = call-poly "Queue_Driver.vi"("State_and_Data_In"=w441, "Error_In"=w443, "Queue_Operation"=w445) -> ("Error_Out"=w446:errorcluster)  [unwired: 10 in, 2 out]
      }
      frame "Exit" {
        w459 = Converter_Operation_Select."Data_to_String"  # Convert_Mode
        w451 = Text_File_Operation_Select."Write"  # INI_Operation_Select
        # "Exit the application"
        n173 = disable-structure shown="Default" {
          disable-tunnel: [w465 w469] -> w462
          frame condition #0 {
            w465 = TRUE  # Stop
            # "Run time mode"
          }
          frame condition #1 (active) {
            w466 = "No"  # Cont
            w467 = "Yes"  # Stop
            w468 = "Do you want to stop execution"  # Message
            # "Developer mode"
            n174 = Two Button Dialog(message=w468, 1:w466, 2:w467) -> (T button?=w469:bool)
          }
        }
        n175 = Generate User Event(user event=w464, event data cluster=w462, error in=w461) -> (user event out=w463:refnum<user-event>, error out=w455:errorcluster)  [unwired: 1 in]
        n176 = call <vilib>:"Set Busy.vi"("error in (no error)"=w455) -> ("error out"=w454:errorcluster)  [unwired: 9 in, 1 out]
        n177 = call "Convert_Class_Data.vi"("I2C_Data"=w458, "Error_In"=w454, "Convert_Mode"=w459) -> ("I2C_Data"=w457:T4, "CSV_String"=w456:string, "Error_Out"=w460:errorcluster)  [unwired: 9 in, 1 out]
        n178 = call "Text_File_Driver.vi"("Data_In"=w456, "Error_Out"=w460, "INI_Operation_Select"=w451) -> ("Error_Out"=w453:errorcluster)  [unwired: 11 in, 1 out]
        n179 = call <vilib>:"Unset Busy.vi"("error in (no error)"=w453) -> ("error out"=w452:errorcluster)  [unwired: 10 in]
      }
    }
  }
  n180 = while {
    tunnel: w18 -> [w475]
    shift-right: [w474] -> w17
    shift-left: w5 -> [w476]
    tunnel: [w472] -> w14
    stop <- w471 stop-if-true
    w473 = 2  # Wait_Time
    # "Producer"
    n181 = event shown="[11] Panel Close?" {
      selector: w475 -> [w477 w480 w489 w498 w505 w514 w523 w532 w541 w550 w557 w560]
      dyn-events: [w477 w480 w489 w498 w505 w514 w523 w532 w541 w550 w557 w560] -> w472
      timeout: w473 -> [_ _ _ _ _ _ _ _ _ _ _ _]
      tunnel: w476 -> [w478 w483 w492 w501 w508 w517 w526 w535 w544 w553 w558 w563]
      tunnel: [w478 w482 w491 w500 w507 w516 w525 w534 w543 w552 w558 w562] -> w474
      tunnel: [_ _ _ _ _ _ _ _ _ _ w556 _] -> w471
      tunnel: T7 {"State"="", "Data"=variant} ("State_and_Data") -> [_ w479 w486 w497 w504 w513 w520 w529 w538 w547 _ w559]
      event Timeout {
        # "Time out happens"
        n182 = event-data() -> ()  [unwired: 1 in, 1 out]
      }
      event "Configure": Value Change {
        w484 = Queue_Operation."Enqueue"  # Queue_Operation
        # "Request to change page"
        n183 = event-data() -> ()  [unwired: 1 in, 1 out]
        n184 = Bundle By Name(cluster=w479, "State"="Change_Page") -> (w481:T7)
        n185 = call-poly "Queue_Driver.vi"("State_and_Data_In"=w481, "Error_In"=w483, "Queue_Operation"=w484) -> ("Error_Out"=w482:errorcluster)  [unwired: 10 in, 2 out]
      }
      event Value Change {
        w493 = Queue_Operation."Enqueue"  # Queue_Operation
        # "Request to select the target"
        n186 = event-data() -> ("NewVal"=w488:T1)  [unwired: 1 in]
        n187 = To Variant(anything=w488) -> (Variant=w487:variant)
        n188 = Bundle By Name(cluster=w486, "State"="Target_Select_Config", "Data"=w487) -> (w490:T7)
        n189 = call-poly "Queue_Driver.vi"("State_and_Data_In"=w490, "Error_In"=w492, "Queue_Operation"=w493) -> ("Error_Out"=w491:errorcluster)  [unwired: 10 in, 2 out]
      }
      event Value Change {
        w496 = TRUE  # Add?
        w502 = Queue_Operation."Enqueue"  # Queue_Operation
        # "Request to add target"
        n190 = event-data() -> ()  [unwired: 1 in, 1 out]
        n191 = To Variant(anything=w496) -> (Variant=w495:variant)
        n192 = Bundle By Name(cluster=w497, "State"="Launch_Add_Targets", "Data"=w495) -> (w499:T7)
        n193 = call-poly "Queue_Driver.vi"("State_and_Data_In"=w499, "Error_In"=w501, "Queue_Operation"=w502) -> ("Error_Out"=w500:errorcluster)  [unwired: 10 in, 2 out]
      }
      event Value Change {
        w509 = Queue_Operation."Enqueue"  # Queue_Operation
        # "Request to delete target"
        n194 = event-data() -> ()  [unwired: 1 in, 1 out]
        n195 = Bundle By Name(cluster=w504, "State"="Delete_Target") -> (w506:T7)
        n196 = call-poly "Queue_Driver.vi"("State_and_Data_In"=w506, "Error_In"=w508, "Queue_Operation"=w509) -> ("Error_Out"=w507:errorcluster)  [unwired: 10 in, 2 out]
      }
      event Value Change {
        w512 = FALSE  # Add?
        w518 = Queue_Operation."Enqueue"  # Queue_Operation
        # "Request to delete target"
        n197 = event-data() -> ()  [unwired: 1 in, 1 out]
        n198 = To Variant(anything=w512) -> (Variant=w511:variant)
        n199 = Bundle By Name(cluster=w513, "State"="Launch_Add_Targets", "Data"=w511) -> (w515:T7)
        n200 = call-poly "Queue_Driver.vi"("State_and_Data_In"=w515, "Error_In"=w517, "Queue_Operation"=w518) -> ("Error_Out"=w516:errorcluster)  [unwired: 10 in, 2 out]
      }
      event Value Change {
        w527 = Queue_Operation."Enqueue"  # Queue_Operation
        # "Request to update the target selected"
        n201 = event-data() -> ("NewVal"=w522:T1)  [unwired: 1 in]
        n202 = To Variant(anything=w522) -> (Variant=w521:variant)
        n203 = Bundle By Name(cluster=w520, "State"="Update_Selected_Target", "Data"=w521) -> (w524:T7)
        n204 = call-poly "Queue_Driver.vi"("State_and_Data_In"=w524, "Error_In"=w526, "Queue_Operation"=w527) -> ("Error_Out"=w525:errorcluster)  [unwired: 10 in, 2 out]
      }
      event Value Change {
        w536 = Queue_Operation."Enqueue"  # Queue_Operation
        # "Request to update the Register selected"
        n205 = event-data() -> ("NewVal"=w531:T1)  [unwired: 1 in]
        n206 = To Variant(anything=w531) -> (Variant=w530:variant)
        n207 = Bundle By Name(cluster=w529, "State"="Update_Selected_Register", "Data"=w530) -> (w533:T7)
        n208 = call-poly "Queue_Driver.vi"("State_and_Data_In"=w533, "Error_In"=w535, "Queue_Operation"=w536) -> ("Error_Out"=w534:errorcluster)  [unwired: 10 in, 2 out]
      }
      event Value Change {
        w545 = Queue_Operation."Enqueue"  # Queue_Operation
        # "Request to update the Mode selected"
        n209 = event-data() -> ()  [unwired: 1 in, 1 out]
        n210 = To Variant(anything="Data Line") -> (Variant=w539:variant)
        n211 = Bundle By Name(cluster=w538, "State"="Generate_Waveform", "Data"=w539) -> (w542:T7)
        n212 = call-poly "Queue_Driver.vi"("State_and_Data_In"=w542, "Error_In"=w544, "Queue_Operation"=w545) -> ("Error_Out"=w543:errorcluster)  [unwired: 10 in, 2 out]
      }
      event Value Change {
        w554 = Queue_Operation."Enqueue"  # Queue_Operation
        # "Request to Hide the Data line"
        n213 = event-data() -> ()  [unwired: 1 in, 1 out]
        n214 = To Variant(anything="Read_Write") -> (Variant=w548:variant)
        n215 = Bundle By Name(cluster=w547, "State"="Hide_Show_Controls", "Data"=w548) -> (w551:T7)
        n216 = call-poly "Queue_Driver.vi"("State_and_Data_In"=w551, "Error_In"=w553, "Queue_Operation"=w554) -> ("Error_Out"=w552:errorcluster)  [unwired: 10 in, 2 out]
      }
      event User Event {
        # "Request to Stop"
        n217 = event-data() -> ("Stop"=w556:bool)  [unwired: 1 in]
      }
      event Panel Close? {
        w564 = Queue_Operation."Enqueue"  # Queue_Operation
        # "Handle panel close"
        n218 = event-data() -> ()  [unwired: 1 in, 1 out]
        n219 = Bundle By Name(cluster=w559, "State"="Exit") -> (w561:T7)
        n220 = call-poly "Queue_Driver.vi"("State_and_Data_In"=w561, "Error_In"=w563, "Queue_Operation"=w564) -> ("Error_Out"=w562:errorcluster)  [unwired: 10 in, 2 out]
        n221 = event-data("Discard?"=TRUE) -> ()  [unwired: 1 in, 1 out]
      }
    }
  }
  n222 = Merge Errors(w17, w16) -> (w15:errorcluster)
  n223 = Unregister For Events(event registration refnum=w14, error in=w15) -> (error out=w13:errorcluster)
  n224 = Destroy User Event(user event=w12, error in=w13) -> (error out=w11:errorcluster)
  n225 = call-poly "Queue_Driver.vi"("Error_In"=w11, "Queue_Operation"=w9) -> ("Error_Out"=w10:errorcluster)  [unwired: 11 in, 2 out]
  n226 = call-poly "Queue_Driver.vi"("Error_In"=w10, "Queue_Operation"=w8) -> ("Error_Out"=→"Error_Out":errorcluster)  [unwired: 11 in, 2 out]
